vi "Get Palette Names.vi"(7 "Run Mode?":bool, 8 "error in (no error)":errorcluster, 9 "Visibility":T1, 10 "3D Comet.lvclass in":refnum<class "3D Comet.lvclass">, 11 "MenuRef":refnum<k9>) -> (0 "error out":errorcluster, 2 "3D Comet.lvclass out":refnum<class "3D Comet.lvclass">, 3 "Dup MenuRef":refnum<k9>)   [LabVIEW 2020, in "3D Comet.lvclass"]
uses:
  <vilib>/Math Plots/3D Math Plots/3D Comet/3D Comet/3D Comet.lvclass
  <vilib>/Math Plots/3D Math Plots/3D Plot/3D Plot/Typedef/Item Visibility.ctl
  <vilib>/Math Plots/3D Math Plots/3D Plot/3D Plot/3D Plot.lvclass
panel:
  in  "Redraw Animation String":string="Play Animation"
  in  "Visibility Item Names":string[](array[string])=["", "Projection Palette"]
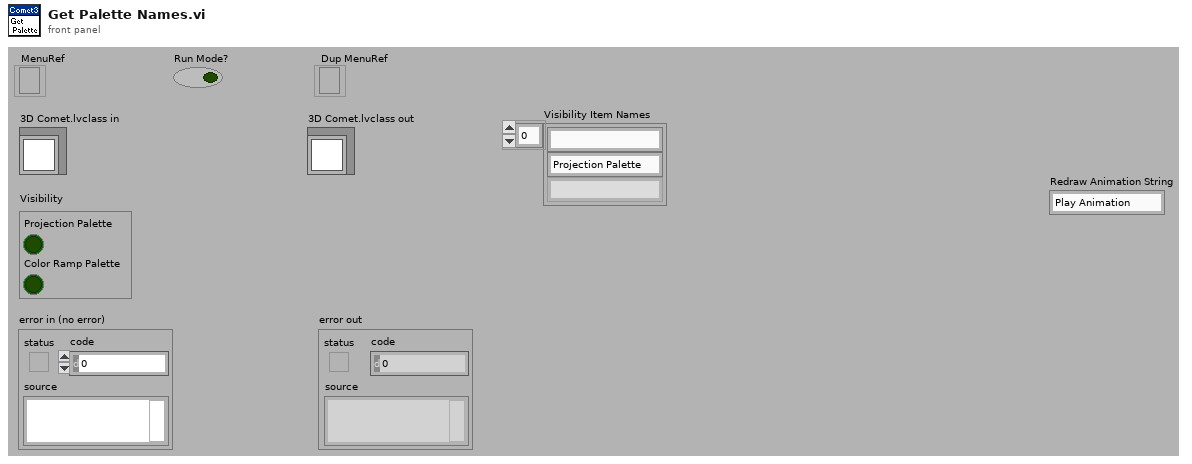
[diagram p1: front panel]
types:
  T1 = typedef "3D Plot.lvclass/Item Visibility.ctl" = cluster{"Projection Palette":bool, "Color Ramp Palette":bool}
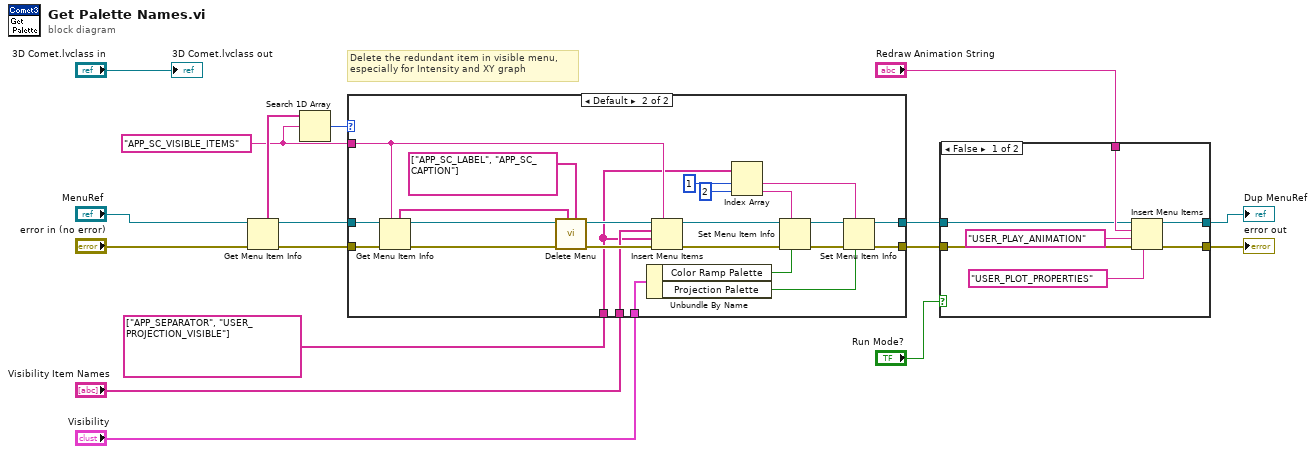
[diagram p0: block diagram]
diagram:
  w11 = "APP_SC_VISIBLE_ITEMS"
  # "Delete the redundant item in visible menu, \nespecially for Intensity and XY graph"
  n1 = Get Menu Item Info(8:"error in (no error)", 11:"MenuRef") -> (0:w15:errorcluster, 3:w13:refnum<k9>, 5:w14:string[])  [unwired: 5 out]
  n2 = Search 1D Array(1D array=w14, element=w11) -> (index of element=w12:i32)  [unwired: 1 out]
  n3 = case shown="Default" w12 {
    tunnel: w13 -> [w19 w43]
    tunnel: [w19 w23] -> w4
    tunnel: w15 -> [w18 w42]
    tunnel: [w18 w20] -> w5
    tunnel: w11 -> [_ w38]
    tunnel: "Visibility" -> [_ w40]
    tunnel: "Visibility Item Names" -> [_ w22]
    tunnel: string[] ["APP_SEPARATOR", "USER_PROJECTION_VISIBLE"] ("item names") -> [_ w21]
    frame -1 {
    }
    frame Default {
      n4 = Get Menu Item Info(7:w38, 8:w42, 11:w43) -> (0:w28:errorcluster, 3:w29:refnum<k9>, 5:w25:string[])  [unwired: 4 out]
      n5 = call <vilib>:"Delete Menu.vi"("Submenu Tags Validated"=string[] ["APP_SC_LABEL", "APP_SC_CAPTION"], "Submenu Tags to Check"=w25, "error in (no error)"=w28, "MenuRef"=w29) -> ("error out"=w26:errorcluster, "Dup MenuRef"=w27:refnum<k9>)  [unwired: 6 in]
      n6 = Unbundle By Name(w40) -> ("Color Ramp Palette"=w31:bool, "Projection Palette"=w30:bool)
      n7 = Insert Menu Items(5:w38, 6:w26, 7:w21, 8:w22, 9:w27) -> (0:w41:errorcluster, 3:w39:refnum<k9>)  [unwired: 2 out]
      n8 = Index Array(array=w21, index #1=1 ("index"), index #2=2 ("index")) -> (element #1=w35:string, element #2=w34:string)
      n9 = Set Menu Item Info(6:w31, 7:w34, 8:w41, 11:w39) -> (0:w37:errorcluster, 3:w36:refnum<k9>)  [unwired: 3 out]
      n10 = Set Menu Item Info(6:w30, 7:w35, 8:w37, 11:w36) -> (0:w20:errorcluster, 3:w23:refnum<k9>)  [unwired: 3 out]
    }
  }
  n11 = case shown="False" "Run Mode?" {
    tunnel: "Redraw Animation String" -> [w48 _]
    tunnel: w5 -> [w47 w51]
    tunnel: w4 -> [w46 w52]
    tunnel: [w45 w52] -> w3
    tunnel: [w44 w51] -> w2
    frame False {
      n12 = Insert Menu Items(4:"USER_PLOT_PROPERTIES" ("menu tag"), 6:w47, 7:"USER_PLAY_ANIMATION", 8:w48, 9:w46) -> (0:w44:errorcluster, 3:w45:refnum<k9>)  [unwired: 2 out]
    }
    frame True {
    }
  }
  "Dup MenuRef" <- w3
  "error out" <- w2
  "3D Comet.lvclass out" <- "3D Comet.lvclass in"
